vi "Validate Scalar Imports.vi"(8 "error in (no error)":errorcluster, 10 "bitfile scalars in":T1[](array[typedef])) -> (0 "error out":errorcluster, 2 "bitfile scalars out":T1[](array[typedef]))   [LabVIEW 2023, in "Scripting API.lvlib"]
uses:
  Scripting API.lvlib
  <userlib>/_OpenG.lib/array/array.llb/openg_array.lvlib
  <userlib>/_OpenG.lib/array/array.llb/Remove Duplicates from 1D Array (String)__ogtk.vi
  TypeDefs/Input Scalar Data.ctl
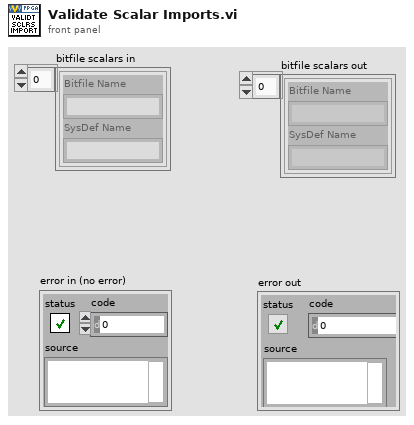
[diagram p1: front panel]
types:
  T1 = typedef "Scripting API.lvlib/Input Scalar Data.ctl" = cluster{"Bitfile Name":string, "SysDef Name":string}
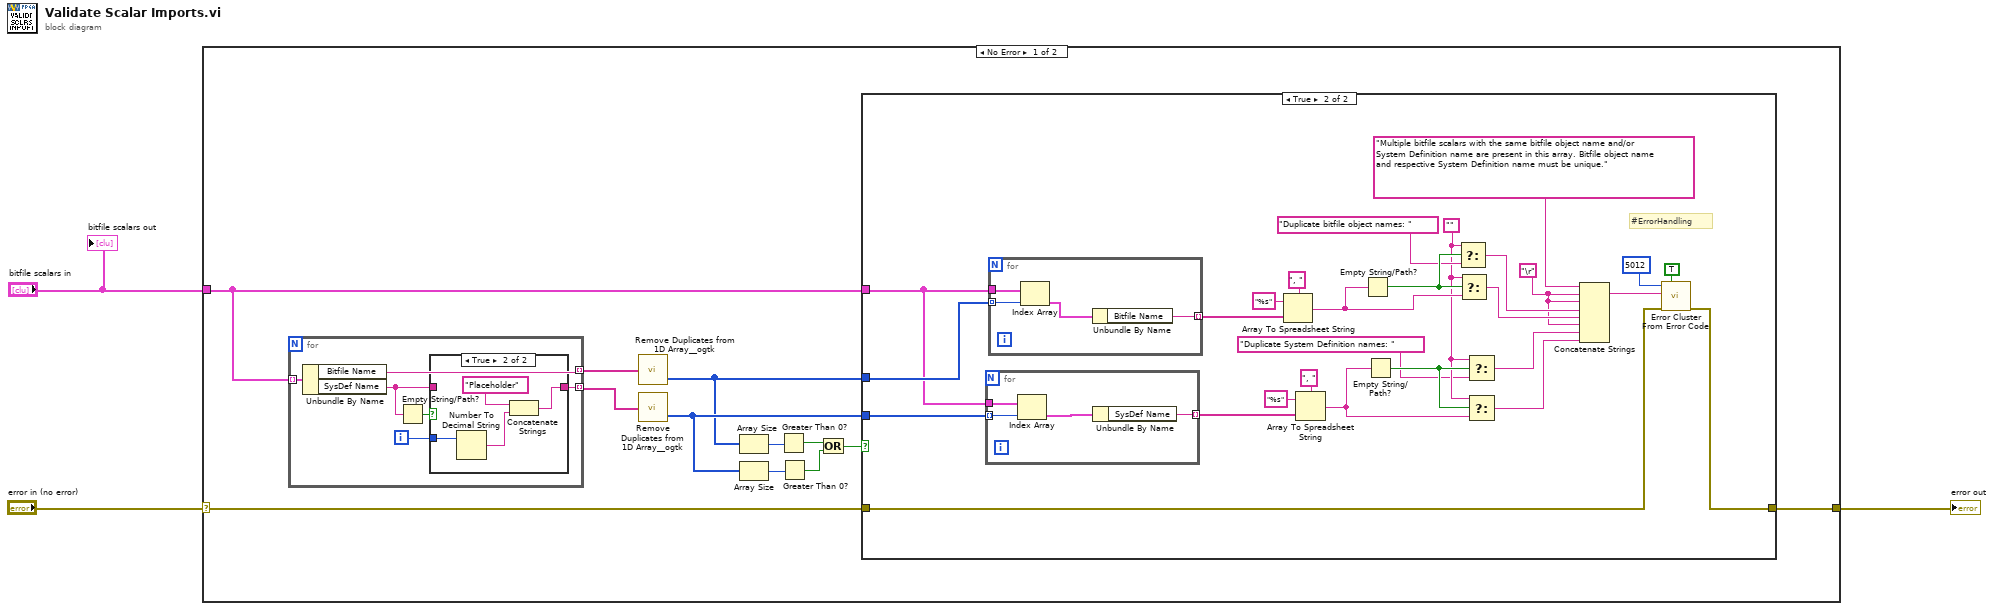
[diagram p0: block diagram]
diagram:
  n1 = case shown="No Error" "error in (no error)" {
    selector: "error in (no error)" -> [w5 w63]
    tunnel: "bitfile scalars in" -> [w12 _]
    tunnel: [w4 w63] -> w1
    frame No Error {
      n2 = for {
        tunnel: w12 -> [w57] mode=indexing
        tunnel: [w56] -> w6 mode=indexing
        tunnel: [w53] -> w13 mode=indexing
        i -> [w52]
        n3 = Unbundle By Name(w57) -> ("Bitfile Name"=w56:string, "SysDef Name"=w54:string)
        n4 = Empty String/Path?(string/path=w54) -> (empty?=w55:bool)
        n5 = case shown="True" w55 {
          tunnel: w54 -> [w58 _]
          tunnel: [w58 w59] -> w53
          tunnel: w52 -> [_ w61]
          frame False {
          }
          frame True {
            n6 = Number To Decimal String(number=w61) -> (decimal integer string=w60:string)  [unwired: 1 in]
            n7 = Concatenate Strings("Placeholder" ("string"), w60) -> (w59:string)
          }
        }
      }
      n8 = call-poly <userlib>:"Remove Duplicates from 1D Array__ogtk.vi"("Input Array"=w6) -> ("indices of removed elements"=w14:i32[])  [unwired: 1 out]
      n9 = call-poly <userlib>:"Remove Duplicates from 1D Array__ogtk.vi"("Input Array"=w13) -> ("indices of removed elements"=w15:i32[])  [unwired: 1 out]
      n10 = Array Size(array=w14) -> (size(s)=w8:i32)
      n11 = Array Size(array=w15) -> (size(s)=w7:i32)
      n12 = Greater Than 0?(x=w8) -> (x > 0?=w9:bool)
      n13 = Greater Than 0?(x=w7) -> (x > 0?=w10:bool)
      n14 = Or(x=w9, y=w10) -> (x .or. y?=w11:bool)
      n15 = case shown="True" w11 {
        tunnel: w12 -> [_ w33]
        tunnel: w14 -> [_ w34]
        tunnel: w15 -> [_ w32]
        tunnel: w5 -> [w16 w39]
        tunnel: [w16 w38] -> w4
        frame False {
        }
        frame True {
          w17 = "\r"
          w22 = ""
          # "#ErrorHandling"
          n16 = for {
            tunnel: w33 -> [w47]
            tunnel: [w45] -> w29 mode=indexing
            tunnel: w32 -> [w44] mode=indexing
            n17 = Index Array(array=w47, index=w44) -> (element=w46:T1)
            n18 = Unbundle By Name(w46) -> ("SysDef Name"=w45:string)
          }
          n19 = for {
            tunnel: w33 -> [w51]
            tunnel: w34 -> [w50] mode=indexing
            tunnel: [w48] -> w35 mode=indexing
            n20 = Index Array(array=w51, index=w50) -> (element=w49:T1)
            n21 = Unbundle By Name(w49) -> ("Bitfile Name"=w48:string)
          }
          n22 = Array To Spreadsheet String(delimiter (Tab)=", ", array=w35, 3:"%s" ("format string")) -> (spreadsheet string=w27:string)
          n23 = Array To Spreadsheet String(delimiter (Tab)=", ", array=w29, 3:"%s" ("format string")) -> (spreadsheet string=w20:string)
          n24 = Empty String/Path?(string/path=w27) -> (empty?=w28:bool)
          n25 = Empty String/Path?(string/path=w20) -> (empty?=w23:bool)
          n26 = Select(t=w22, s=w28, f="Duplicate bitfile object names: " ("string")) -> (s? t:f=w25:string)
          n27 = Select(t=w22, s=w28, f=w27) -> (s? t:f=w24:string)
          n28 = Select(t=w22, s=w23, f="Duplicate System Definition names: " ("string")) -> (s? t:f=w19:string)
          n29 = Select(t=w22, s=w23, f=w20) -> (s? t:f=w18:string)
          n30 = Concatenate Strings("Multiple bitfile scalars with the same bitfile object name and/or System Definition name are present in this array. Bitfile object name and respective System Definition name must be unique." ("error message (\"\")"), w17, w17, w25, w24, w17, w19, w18) -> (w41:string)
          n31 = call <vilib>:"Error Cluster From Error Code.vi"("show call chain? (False)"=TRUE, "error in (no error)"=w39, "error message (\"\")"=w41, "error code (0)"=5012) -> ("error out"=w38:errorcluster)  [unwired: 5 in]
        }
      }
    }
    frame Error {
    }
  }
  "error out" <- w1
  "bitfile scalars out" <- "bitfile scalars in"
